vi "String Unescape.vi"(11 "Escaped String":string) -> (3 "Unescaped String":string)   [LabVIEW 2022 SP3, in "LabVIEW-Config.lvlib"]
uses:
  LabVIEW-Config.lvlib
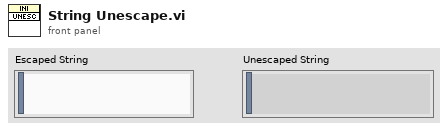
[diagram p1: front panel]
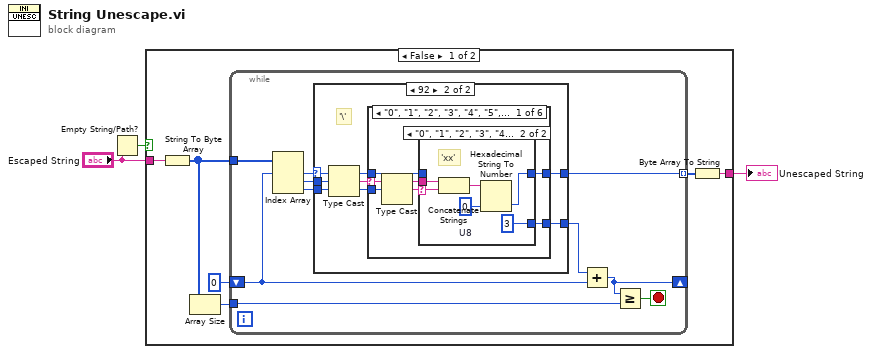
[diagram p0: block diagram]
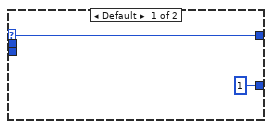
[diagram p2: hidden frame]
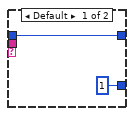
[diagram p3: hidden frame]
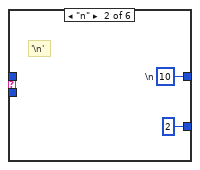
[diagram p4: hidden frame]
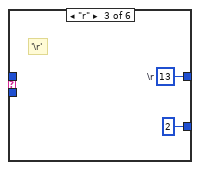
[diagram p5: hidden frame]
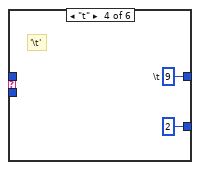
[diagram p6: hidden frame]
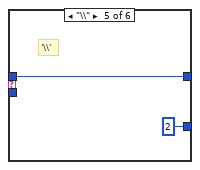
[diagram p7: hidden frame]
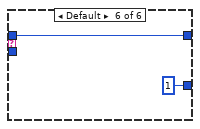
[diagram p8: hidden frame]
diagram:
  n1 = Empty String/Path?(string/path="Escaped String") -> (empty?=w1:bool)
  n2 = case shown="False" w1 {
    tunnel: "Escaped String" -> [w9 w52]
    tunnel: [w5 w52] -> w3
    frame False {
      n3 = String To Byte Array(string=w9) -> (unsigned byte array=w7:u8[])
      n4 = Array Size(array=w7) -> (size(s)=w6:i32)
      n5 = while {
        tunnel: w7 -> [w19]
        shift-right: [w14] -> _
        shift-left: 0 -> [w15]
        tunnel: w6 -> [w11]
        tunnel: [w10] -> w4 mode=indexing
        stop <- w12 stop-if-true
        n6 = Index Array(array=w19, index #1=w15) -> (element #1=w18:u8, element #2=w17:u8, element #3=w16:u8)  [unwired: 2 in]
        n7 = case shown="92" w18 {
          selector: w18 -> [w21 w26]
          tunnel: w17 -> [_ w27]
          tunnel: w16 -> [_ w22]
          tunnel: [w21 w25] -> w10
          tunnel: [1 w24] -> w13
          frame Default {
          }
          frame 92 {
            # "'\\'"
            n8 = Type Cast(x=w27) -> (*(type *) &x=w23:string)  [unwired: 1 in]
            n9 = case shown="\"0\", \"1\", \"2\", \"3\", \"4\", \"5\", \"6\", \"7\", \"8\", \"9\", \"A\", \"B\", \"C\", \"D\", \"E\", \"F\"" w23 {
              selector: w23 -> [w32 _ _ _ _ _]
              tunnel: w26 -> [w29 _ _ _ w49 w51]
              tunnel: [w30 w43 w45 w47 w49 w51] -> w25
              tunnel: [w28 2 2 2 2 1] -> w24
              tunnel: w22 -> [w33 _ _ _ _ _]
              frame "0", "1", "2", "3", "4", "5", "6", "7", "8", "9", "A", "B", "C", "D", "E", "F" {
                n10 = Type Cast(x=w33) -> (*(type *) &x=w31:string)  [unwired: 1 in]
                n11 = case shown="\"0\", \"1\", \"2\", \"3\", \"4\", \"5\", \"6\", \"7\", \"8\", \"9\", \"A\", \"B\", \"C\", \"D\", \"E\", \"F\"" w31 {
                  selector: w31 -> [_ w40]
                  tunnel: w32 -> [_ w41]
                  tunnel: [w35 w37] -> w30
                  tunnel: w29 -> [w35 _]
                  tunnel: [1 3] -> w28
                  frame Default {
                  }
                  frame "0", "1", "2", "3", "4", "5", "6", "7", "8", "9", "A", "B", "C", "D", "E", "F" {
                    w38 = u8 0  # U8
                    # "'xx'"
                    n12 = Concatenate Strings(w41, w40) -> (w39:string)
                    n13 = Hexadecimal String To Number(string=w39, default (0uL)=w38) -> (number=w37:u8)  [unwired: 1 in, 1 out]
                  }
                }
              }
              frame "n" {
                w43 = u8 10  # \n
                # "'\\n'"
              }
              frame "r" {
                w45 = u8 13  # \r
                # "'\\r'"
              }
              frame "t" {
                w47 = u8 9  # \t
                # "'\\t'"
              }
              frame "\\" {
                # "'\\\\'"
              }
              frame Default {
              }
            }
          }
        }
        n14 = Add(x=w13, y=w15) -> (x+y=w14:i32)
        n15 = Greater Or Equal?(x=w14, y=w11) -> (x >= y?=w12:bool)
      }
      n16 = Byte Array To String(unsigned byte array=w4) -> (string=w5:string)
    }
    frame True {
    }
  }
  "Unescaped String" <- w3
